vi "Set Version.vi"(8 "error in":errorcluster, 10 "XML Node":refnum<k20>, 11 "Custom Device Config Ref in":refnum<data-value>) -> (0 "error out":errorcluster, 3 "Custom Device Config Ref out":refnum<data-value>)   [LabVIEW 2024, in "Config File Parser.lvlib" / "Custom Device Config.lvclass"]
uses:
  Custom Device Config.lvclass
  Custom Device Config.lvclass/Custom Device Config.ctl
  <vilib>/xml/Close Reference(Node).vi
  <vilib>/xml/NI_XML.lvlib
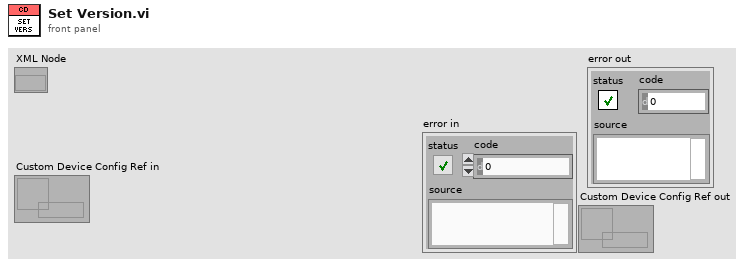
[diagram p1: front panel]
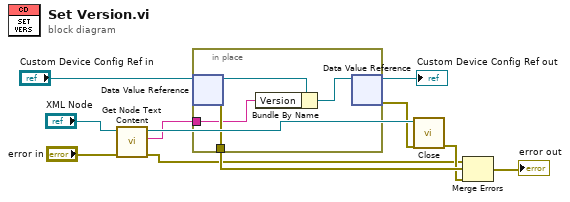
[diagram p0: block diagram]
diagram:
  n1 = call <vilib>:"Get Node Text Content.vi"("error in (no error)"="error in", "node in"="XML Node") -> ("error out"=w3:errorcluster, "node text"=w4:string, "node out"=w10:refnum<k20>)  [unwired: 7 in]
  n2 = in-place "In Place Element Structure" {
    in-place-border: [w13] -> w8
    in-place-border: w4 -> [w12]
    n3 = in-place-dvr #1("Custom Device Config Ref in") -> (w15:refnum<class "Custom Device Config.lvclass">, w13:errorcluster)
    n4 = Bundle By Name(cluster=w15, "Version"=w12) -> (w14:refnum<class "Custom Device Config.lvclass">)
    n5 = in-place-dvr #1(w14) -> (→"Custom Device Config Ref out":refnum<data-value>, w9:errorcluster)
  }
  n6 = call-poly <vilib>:"Close.vi"("error in (no error)"=w9, "node"=w10) -> ("error out"=w7:errorcluster)  [unwired: 7 in]
  n7 = Merge Errors(w3, w8, w7) -> (→"error out":errorcluster)
